vi "Substitute Actor.vi"(10 "Substitute Actor in":refnum<class "Actor.lvclass">, 11 "Current Engine":refnum<class "Engine.lvclass">) -> (0 "error out":errorcluster, 2 "Substitute Actor out":refnum<class "Actor.lvclass">)   [LabVIEW 2019, in "Engine.lvlib" / "Engine.lvclass"]
doc: "This method copies information from the <b>Current Actor</b> to the <b>Substitute Actor</b>, including the to-self and the to-caller queue references. The purpose of this function is to allow an actor to define a method that replaces itself with another actor, useful for implementing a State Pattern Actor. Child classes should override this method to copy any additional fields that they need from the current to the substitute.\n\nThis method may return error code 678010: Illegal substitution. Overrides of this method may choose to return this error if the new actor is not one that is an appropriate substitute for the current actor, for whatever standards of \"appropriate\" are chosen for the current actor. If returning an error, override VIs should return the unmodified <b>Current Actor</b> as <b>Substitute Actor out</b>."
uses:
  Project/Engine.lvclass
  C:/Users/Public/Documents/Development/builds/Engine/Actor Framework.lvlibp/1abvi3w/vi.lib/ActorFramework/Actor/Actor.lvclass
  builds/Engine/Actor Framework.lvlibp/1abvi3w/vi.lib/ActorFramework/Actor/Actor.lvclass
  Project/Engine.lvclass/Engine.ctl
  builds/Engine/State Actor.lvlibp/Library/State Actor.lvclass
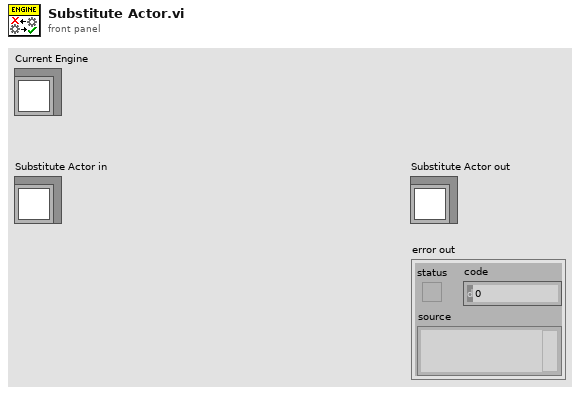
[diagram p1: front panel]
types:
  T1 = typedef "Engine.lvlib/Engine.lvclass/Engine Events.ctl" = cluster{"System Event":T2, "Manual":T3, "UUT":T4, "Interface Events":T5}
  T2 = typedef "Engine.lvlib/Engine.lvclass/System Events.ctl" = cluster{"Fault Event":refnum<user-event>, "SystemStatus Event":refnum<user-event>, "Automation":refnum<user-event>}
  T3 = typedef "Engine.lvlib/Engine.lvclass/Manual Events.ctl" = cluster{"QuickStart Event":refnum<user-event>, "SafeBTE Event":refnum<user-event>, "TogglePower Event":refnum<user-event>, "Change Instrument Event":refnum<user-event>, "Toggle Launch Event":refnum<user-event>, "UUTSupply":refnum<user-event>}
  T4 = typedef "Engine.lvlib/Engine.lvclass/UUT_Events.ctl" = cluster{"UUT_Name":refnum<user-event>, "Test_Name":refnum<user-event>, "Test_Operator":refnum<user-event>, "Test_Witness":refnum<user-event>, "Pedigree_Event":refnum<user-event>}
  T5 = typedef "Engine.lvlib/Engine.lvclass/Interface Events.ctl" = cluster{"Interface_Command":refnum<user-event>, "Telemetry_Descriptor":refnum<user-event>, "AsynchTLM_Descriptor":refnum<user-event>}
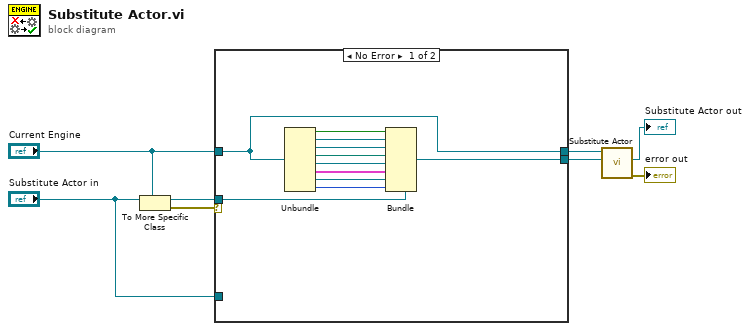
[diagram p0: block diagram]
diagram:
  n1 = To More Specific Class(target class="Current Engine", reference="Substitute Actor in") -> (specific class reference=w5:refnum<class "Engine.lvclass">, error out=w6:errorcluster)  [unwired: 1 in]
  n2 = case shown="No Error" w6 {
    tunnel: w5 -> [w19 _]
    tunnel: "Substitute Actor in" -> [_ w21]
    tunnel: [w10 w21] -> w3
    tunnel: "Current Engine" -> [w9 w20]
    tunnel: [w9 w20] -> w1
    frame No Error {
      n3 = Unbundle(w9) -> (w18:bool, w17:refnum<class "Message Enqueuer.lvclass">, w16:refnum<class "Message Enqueuer.lvclass">, w15:path, w14:refnum<vi>, w13:T1, w12:refnum<class "QDMH.lvclass">, w11:enum16{"STAT", "BB", "PT", "EM", "FT"})
      n4 = Bundle(cluster=w19, w18, w17, w16, w15, w14, w13, w12, w11) -> (w10:refnum<class "Engine.lvclass">)
    }
    frame Error {
    }
  }
  n5 = call-parent "Substitute Actor.vi"("Substitute Actor in"=w3, "Current Panel Actor"=w1) -> ("error out"=→"error out":errorcluster, "Substitute Actor out"=→"Substitute Actor out":refnum<class "Actor.lvclass">)  [unwired: 8 in]
